vi "New Abstract Group.vi"(8 "error in (no error)":errorcluster, 10 "Group Config":refnum<class "Group Config.lvclass">, 11 "ChannelService in":refnum<class "ChannelService.lvclass">) -> (0 "error out":errorcluster, 2 "Group":refnum<class "Group.lvclass">, 3 "ChannelService out":refnum<class "ChannelService.lvclass">)   [LabVIEW 2020, in "Vecto.lvlib" / "ChannelService.lvclass"]
uses:
  ChannelService.lvclass
  Group Config/Group Config.lvclass
  Group/Group.lvclass
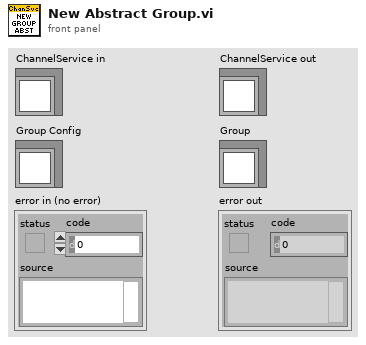
[diagram p1: front panel]
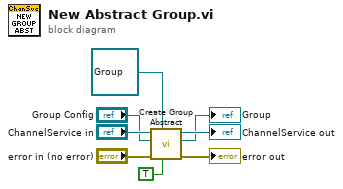
[diagram p0: block diagram]
diagram:
  n1 = call "Create Group Abstract.vi"("Skip Type Check (F)"=TRUE, "Group Type"=refnum<class "Group.lvclass"> refnum ("Vecto.lvlib:GroupAbstract.lvclass"), "error in (no error)"="error in (no error)", "Group Config"="Group Config", "ChannelService in"="ChannelService in") -> ("error out"=→"error out":errorcluster, "Group"=→"Group":refnum<class "Group.lvclass">, "ChannelService out"=→"ChannelService out":refnum<class "ChannelService.lvclass">)  [unwired: 4 in]
